vi "Exchange for Access Token.vi"(8 "error in (no error)":errorcluster, 9 "OAuth Credentials (request)":T1={"Consumer Key"="", "Signature Method"=enum."HMAC-SHA1", "Token"="", "Version"="", "Token Secret"="", "Consumer Secret"=""}, 10 "Pin":string, 11 "Access Request URL":string) -> (0 "error out":errorcluster, 1 "OAuth Credentials (access)":T1={"Consumer Key"="", "Signature Method"=enum."HMAC-SHA1", "Token"="", "Version"="", "Token Secret"="", "Consumer Secret"=""}, 2 "body":string, 3 "headers":string)   [LabVIEW 2011, in "i3-oauth.lvlib"]
doc: "Uses a PIN to exchange an OAuth request token and token secret for an OAuth access token and token secret."
uses:
  i3-oauth.lvlib
  Controls/OAuth Credentials.ctl
  Controls/Signature Method.ctl
  Controls/HTTP Method.ctl
  <vilib>/httpClient/POSTBuffer.vi
  <vilib>/httpClient/LabVIEWHTTPClient.lvlib
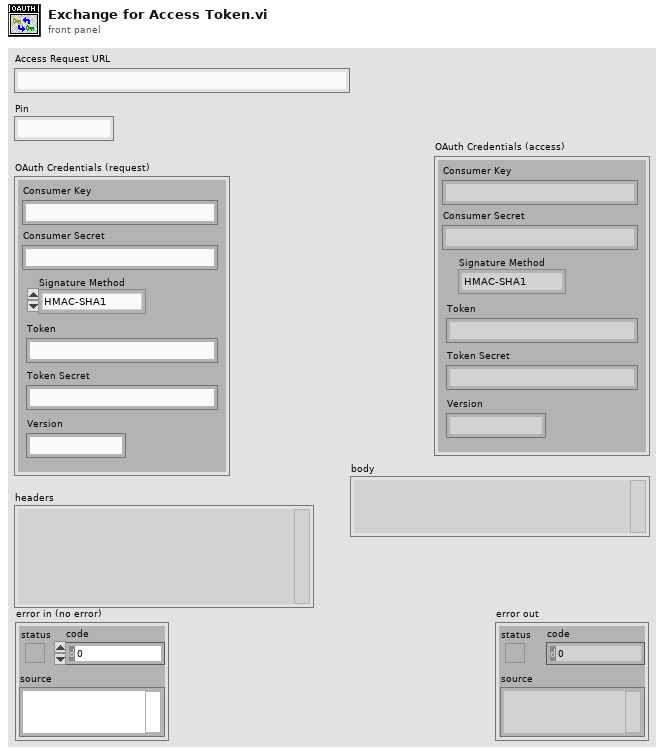
[diagram p1: front panel]
types:
  T1 = typedef "i3-oauth.lvlib/OAuth Credentials.ctl" = cluster{"Consumer Key":string, "Signature Method":T2, "Token":string, "Version":string, "Token Secret":string, "Consumer Secret":string}
  T2 = typedef "i3-oauth.lvlib/Signature Method.ctl" = enum16{"HMAC-MD5", "HMAC-SHA1", "HMAC-SHA224", "HMAC-SHA256", "HMAC-SHA384", "HMAC-SHA512"}
  T3 = typedef "i3-oauth.lvlib/HTTP Method.ctl" = enum16{"GET", "POST", "PUT", "DELETE"}
  T4 = typedef "LabVIEWHTTPClient.lvlib/ClientHandle.ctl" = refnum<k1>
  T5 = typedef "i3-oauth.lvlib/key-value-pairs.ctl" = cluster{"key":string, "value":string}
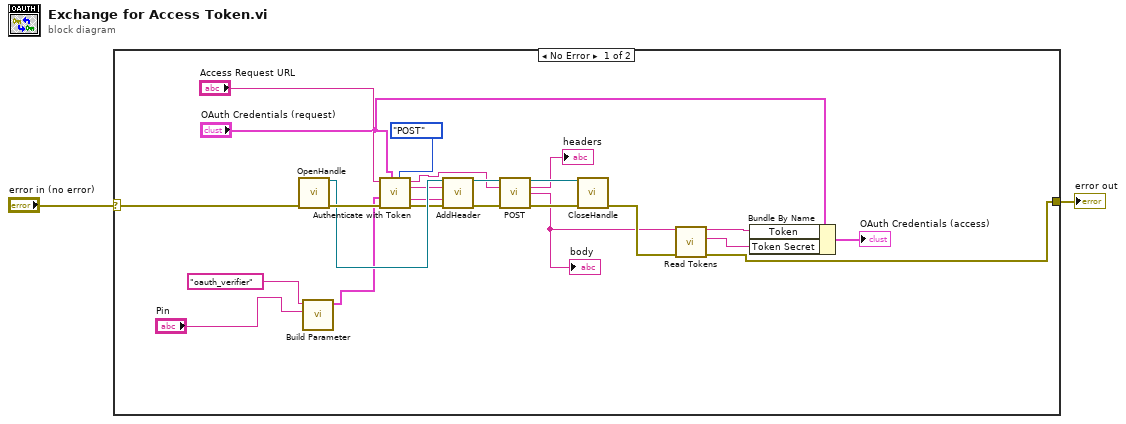
[diagram p0: block diagram]
diagram:
  n1 = case shown="No Error" "error in (no error)" {
    selector: "error in (no error)" -> [w22 w27]
    tunnel: [w3 w27] -> w1
    frame No Error {
      n2 = call <vilib>:"OpenHandle.vi"("error in (no error)"=w22) -> ("client handle out"=w11:T4, "error out"=w26:errorcluster)  [unwired: 13 in]
      n3 = call "Build Parameter.vi"("Value"="Pin", "Key"="oauth_verifier" ("key")) -> ("Parameter Array"=w5:T5[])  [unwired: 9 in]
      n4 = call "Authenticate with Token.vi"("HTTP Method"=HTTP_Method."POST", "OAuth Credentials"="OAuth Credentials (request)", "error in (no error)"=w26, "Header Parameters"=w5, "Base URL"="Access Request URL") -> ("error out"=w8:errorcluster, "Header Value"=w9:string, "Header Parameter"=w10:string, "Full URL"=w6:string)  [unwired: 2 in, 1 out]
      n5 = call <vilib>:"AddHeader.vi"("client handle"=w11, "header"=w10, "value"=w9, "error in (no error)"=w8) -> ("client handle out"=w12:T4, "error out"=w7:errorcluster)  [unwired: 10 in]
      n6 = call-poly <vilib>:"POST.vi"("client handle"=w12, "url"=w6, "error in (no error)"=w7) -> ("client handle out"=w24:T4, "headers"=→"headers":string, "body"=w17:string, "error out"=w25:errorcluster)  [unwired: 9 in]
      "body" <- w17
      n7 = call <vilib>:"CloseHandle.vi"("client handle"=w24, "error in (no error)"=w25) -> ("error out"=w20:errorcluster)  [unwired: 13 in]
      n8 = call "Read Tokens.vi"("error in (no error)"=w20, "input string"=w17) -> ("error out"=w3:errorcluster, "Token Secret"=w18:string, "Token"=w19:string)  [unwired: 7 in]
      n9 = Bundle By Name(cluster="OAuth Credentials (request)", "Token"=w19, "Token Secret"=w18) -> (→"OAuth Credentials (access)":T1)
    }
    frame Error {
    }
  }
  "error out" <- w1
